vi "4072_Global.vi"() -> ()   [LabVIEW 2010, in "NI PXI-4072 DMM Custom Device.lvlib"]
uses:
  NI PXI-4072 DMM Custom Device.lvlib
panel:
  in  "Resistance Enum":string="Resistance Enum"
  in  "Capacitance Enum":string="Capacitance Enum"
  in  "Voltage Enum":string="Voltage Enum"
  in  "Processor":string="Processor"
  in  "Resolution (Digits)":string="Resolution (Digits)"
  in  "Range":string="Range"
  in  "Measurement Type":string="Measurement Type"
  in  "Device Name":string="Device Name"
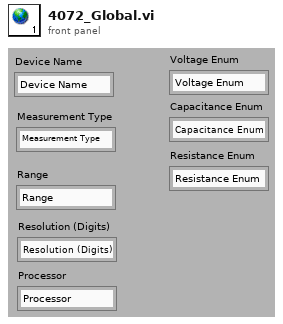
[diagram p1: front panel]
diagram:
